vi "Test Throwing Error.vi"(8 "error in (no error)":errorcluster, 11 "LUnit Setup Error in":refnum<class "LUnit Setup Error.lvclass">) -> (0 "error out":errorcluster, 3 "LUnit Setup Error out":refnum<class "LUnit Setup Error.lvclass">)   [LabVIEW 2020, in "LUnit Setup Error.lvclass"]
uses:
  LUnit Setup Error.lvclass
  C:/Program Files (x86)/National Instruments/LabVIEW 2020/vi.lib/Astemes/LUnit/Test Case.lvclass
  <vilib>/Astemes/LUnit/Test Case.lvclass/Test Case.ctl
  <vilib>/Astemes/LUnit/Append Pass Result.vi
  <vilib>/Astemes/LUnit/Run In UI.vi
  <vilib>/Utility/error.llb/Clear Errors.vi
  <vilib>/Astemes/LUnit/Test Case.lvclass
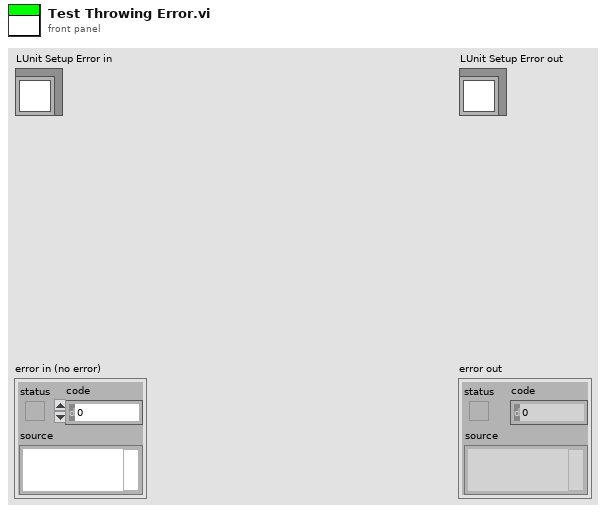
[diagram p1: front panel]
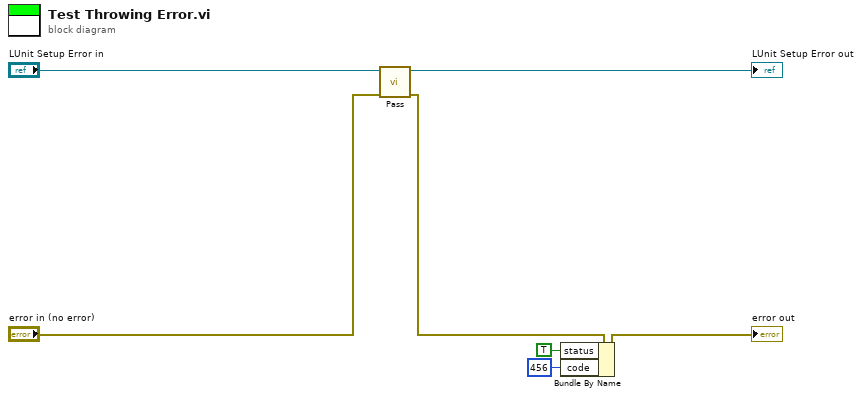
[diagram p0: block diagram]
diagram:
  n1 = call <vilib>:"Pass.vi"("error in (no error)"="error in (no error)", "LUnit Test Case In"="LUnit Setup Error in") -> ("error out"=w1:errorcluster, "LUnit Test Case Out"=→"LUnit Setup Error out":refnum<class "LUnit Setup Error.lvclass">)  [unwired: 8 in]
  n2 = Bundle By Name(cluster=w1, "status"=TRUE, "code"=456) -> (→"error out":errorcluster)
